vi "Weather Station UI.vi"() -> ()   [LabVIEW 2019]
uses:
  <vilib>/DAQmx/create/channels.llb/DAQmx Create Channel (AI-Temperature-Thermocouple).vi
panel:
  out "Temperature History":dbl(graph)
  in  "Stop":bool
  out "Warning":string
  in  "Lower Limit":dbl=20.0
  in  "Upper Limit":dbl=30.0
  in  "Thermocouple Channel":tag="PCI-6221/ai0"
  # "Temperature Ranges (deg C)"
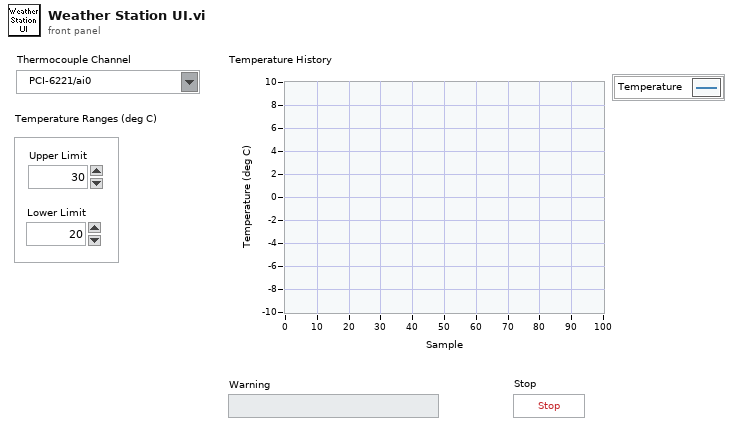
[diagram p1: front panel]
types:
  T1 = enum16{"open", "replace", "create", "open or create", "replace or create", "replace or create with confirmation"}
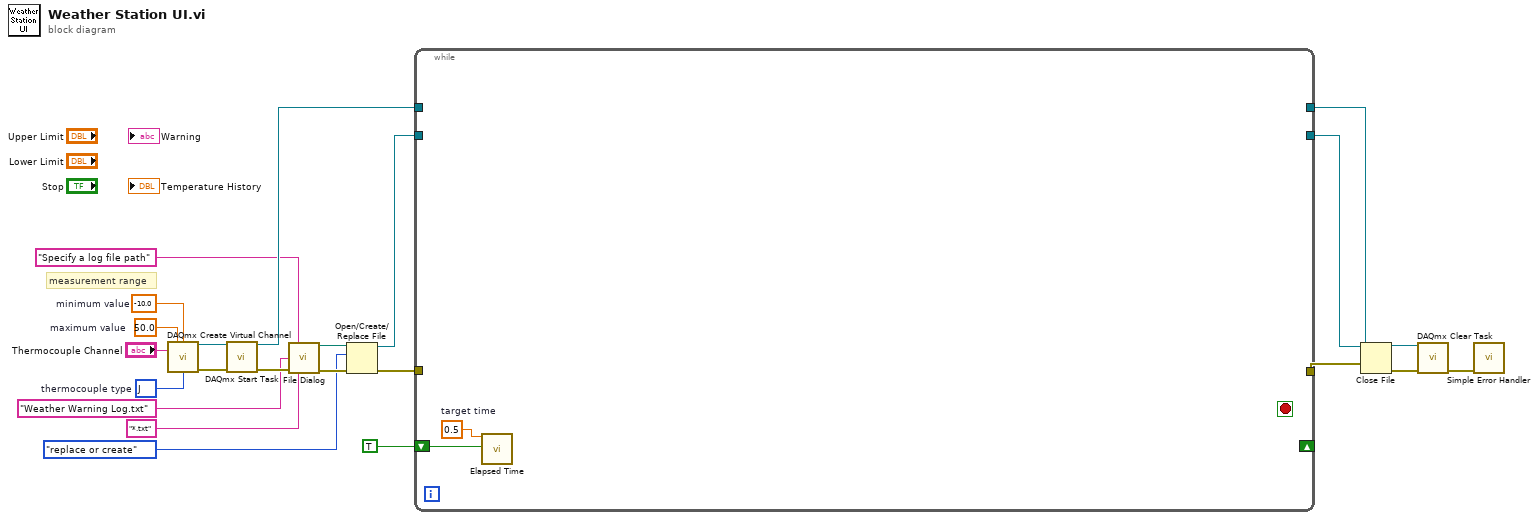
[diagram p0: block diagram]
diagram:
  w20 = 10072 items=["J"=10072, "K"=10073, "N"=10077, "R"=10082, "S"=10085, "T"=10086, "B"=10047, "E"=10055]  # thermocouple type
  w21 = -10.0  # minimum value
  w22 = 50.0  # maximum value
  # "measurement range"
  n1 = call-poly <vilib>:"DAQmx Create Virtual Channel.vi"("maximum value"=w22, "minimum value"=w21, "physical channels"="Thermocouple Channel", "thermocouple type"=w20) -> ("task out"=w19:refnum<k21>, "error out"=w18:errorcluster)  [unwired: 10 in]
  n2 = call <vilib>:"DAQmx Start Task.vi"("task/channels in"=w19, "error in"=w18) -> ("task out"=w14:refnum<k21>, "error out"=w9:errorcluster)  [unwired: 12 in]
  n3 = call "File Dialog"("prompt"="Specify a log file path", "default name"="Weather Warning Log.txt", "error in"=w9, "pattern (all files)"="*.txt") -> ("selected path"=w16:path, "error out"=w17:errorcluster)  [unwired: 8 in, 2 out]
  n4 = Open/Create/Replace File(file path (use dialog)=w16, error in=w17, operation (0:open)=T1."replace or create") -> (refnum out=w15:refnum<file>, error out=w13:errorcluster)  [unwired: 3 in, 1 out]
  n5 = while {
    tunnel: w15 -> [_]
    tunnel: w14 -> [_]
    tunnel: w13 -> [_]
    shift-right: _ -> [_]
    shift-left: TRUE -> [w23]
    tunnel: [_] -> w4
    tunnel: [_] -> w3
    tunnel: [_] -> w5
    stop <- _ stop-if-true
    w24 = 0.5  # target time
    n6 = call "Elapsed Time"("Time Target (s)"=w24, "Reset"=w23) -> ()  [unwired: 10 in, 8 out]
  }
  n7 = Close File(refnum=w5, error in=w3) -> (error out=w11:errorcluster)  [unwired: 1 out]
  n8 = call <vilib>:"DAQmx Clear Task.vi"("task in"=w4, "error in"=w11) -> ("error out"=w10:errorcluster)  [unwired: 13 in]
  n9 = call <vilib>:"Simple Error Handler.vi"("error in (no error)"=w10) -> ()  [unwired: 4 in, 5 out]
